vi "TLPM_PowerMeter.vi"() -> ()   [LabVIEW 2014]
panel:
  in  "Average Time (0.0)":dbl=0.05
  out "Active":bool
  in  "stop":bool
  out "Power Value":dbl=0.000114588314 caption="Optical Power [W]" format="%#_4p"
  # "TLPM"
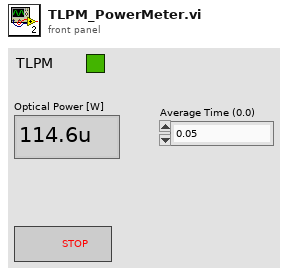
[diagram p1: front panel]
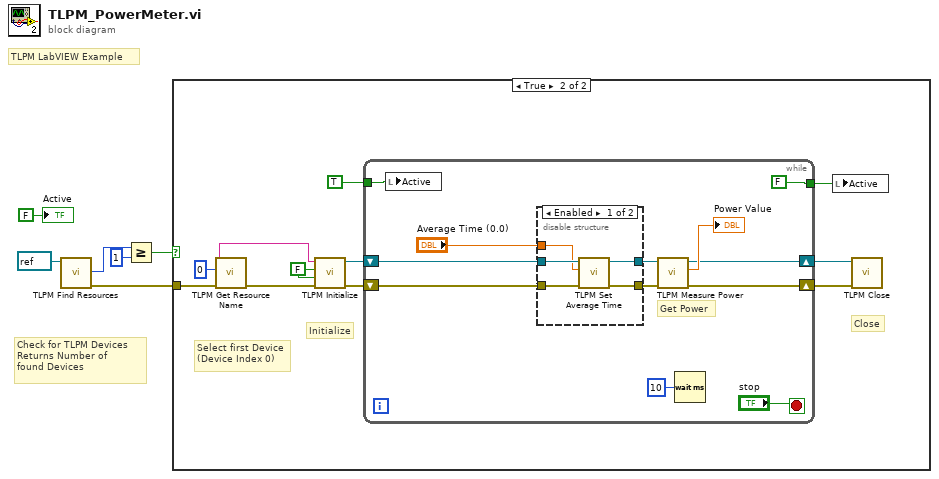
[diagram p0: block diagram]
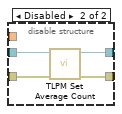
[diagram p3: hidden frame]
diagram:
  # "TLPM LabVIEW Example"
  # "Check for TLPM Devices\nReturns Number of\nfound Devices"
  n1 = call "TLPM Find Resources.vi"("instrument handle"=refnum<visa-resource-name> refnum) -> ("error out"=w5:errorcluster, "Resource Count"=w3:u32)  [unwired: 8 in, 1 out]
  n2 = Greater Or Equal?(x=w3, y=u32 1) -> (x >= y?=w4:bool)
  n3 = case shown="True" w4 {
    tunnel: w5 -> [_ w13]
    frame False {
    }
    frame True {
      w11 = FALSE ("ID Query (Do Query)")
      # "Close"
      # "Initialize"
      # "Select first Device\n(Device Index 0)"
      n4 = call "TLPM Get Resource Name.vi"("error in (no error)"=w13, "Index (0)"=u32 0 ("Device Index")) -> ("error out"=w16:errorcluster, "Resource Name"=w14:string)  [unwired: 7 in, 1 out]
      n5 = call "TLPM Initialize.vi"("error in (no error)"=w16, "Reset Device (Reset Device)"=w11, "ID Query (Do Query)"=w11, "resource name"=w14) -> ("error out"=w9:errorcluster, "instrument handle out"=w10:refnum<visa-resource-name>)  [unwired: 6 in]
      n6 = while {
        shift-right: [w24] -> w17
        shift-left: w10 -> [w22]
        shift-right: [w23] -> w15
        shift-left: w9 -> [w21]
        tunnel: [FALSE ("Active")] -> w8
        tunnel: TRUE ("Active") -> [w25]
        stop <- "stop" stop-if-true
        # "Get Power"
        n7 = local write "Active"(w25) -> ()
        n8 = disable-structure shown="Enabled" {
          disable-tunnel: w22 -> [w34 w38]
          disable-tunnel: w21 -> [w33 w36]
          disable-tunnel: [w32 w37] -> w20
          disable-tunnel: [w31 w35] -> w19
          disable-tunnel: "Average Time (0.0)" -> [w30 _]
          frame Enabled {
            n9 = call "TLPM Set Average Time.vi"("error in (no error)"=w33, "Average Time (0.0)"=w30, "instrument handle"=w34) -> ("error out"=w31:errorcluster, "instrument handle out"=w32:refnum<visa-resource-name>)  [unwired: 7 in]
          }
          frame Disabled {
            n10 = call "TLPM Set Average Count.vi"("error in (no error)"=w36, "instrument handle"=w38) -> ("error out"=w35:errorcluster, "instrument handle out"=w37:refnum<visa-resource-name>)  [unwired: 8 in]
          }
        }
        n11 = call "TLPM Measure Power.vi"("error in (no error)"=w19, "instrument handle"=w20) -> ("error out"=w23:errorcluster, "Power"=→"Power Value":dbl, "instrument handle out"=w24:refnum<visa-resource-name>)  [unwired: 7 in]
        n12 = Wait (ms)(milliseconds to wait=u32 10) -> ()  [unwired: 1 out]
      }
      n13 = local write "Active"(w8) -> ()
      n14 = call "TLPM Close.vi"("error in (no error)"=w15, "instrument handle"=w17) -> ()  [unwired: 9 in, 1 out]
    }
  }
  "Active" <- FALSE ("Active")
